vi "Ctor.vi"(8 "error in (no error)":errorcluster, 10 "Object":refnum<class>) -> (0 "error out":errorcluster, 3 "ClassReflector out":refnum<class "ClassReflector.lvclass">)   [LabVIEW 2023, in "ClassReflector.lvclass"]
uses:
  ClassReflector.lvclass
  ClassReflector.lvclass/ClassReflector.ctl
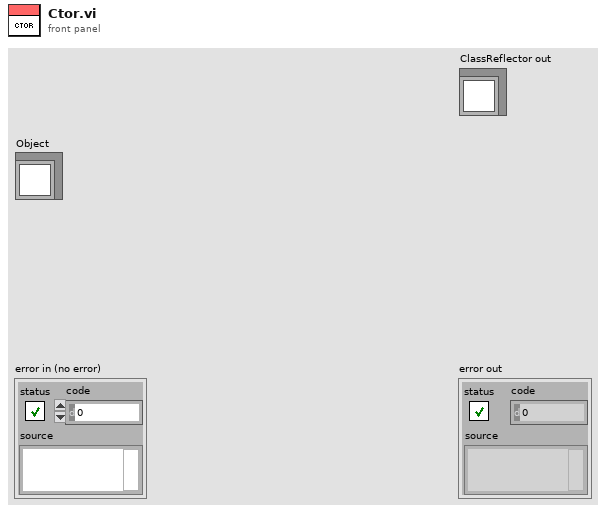
[diagram p1: front panel]
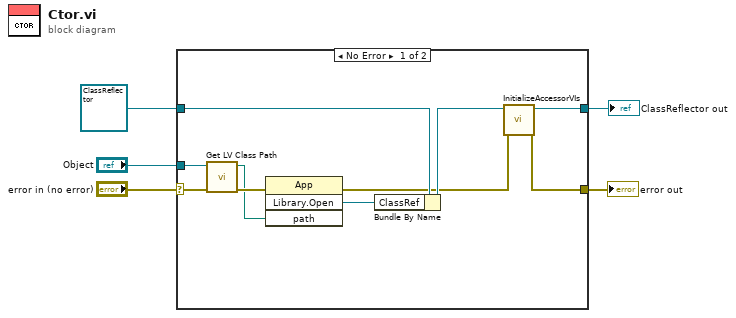
[diagram p0: block diagram]
diagram:
  n1 = case shown="No Error" "error in (no error)" {
    selector: "error in (no error)" -> [w15 w17]
    tunnel: [w6 w17] -> w4
    tunnel: [w8 w16] -> w2
    tunnel: refnum<class "ClassReflector.lvclass"> refnum ("ClassReflector in") -> [w11 w16]
    tunnel: "Object" -> [w13 _]
    frame No Error {
      n2 = call <vilib>:"Get LV Class Path.vi"("error in (no error)"=w15, "object"=w13) -> ("error out"=w14:errorcluster, "class path"=w12:path)  [unwired: 8 in]
      n3 = invoke class="App" method="Library.Open"(error in=w14, "path"=w12) -> (error out=w7:errorcluster, "Open Library"=w10:refnum<vi>)  [unwired: 2 in, 2 out]
      n4 = Bundle By Name(cluster=w11, "ClassRef"=w10) -> (w9:refnum<class "ClassReflector.lvclass">)
      n5 = call "InitializeAccessorVIs.vi"("error in (no error)"=w7, "ClassReflector in"=w9) -> ("error out"=w6:errorcluster, "ClassReflector out"=w8:refnum<class "ClassReflector.lvclass">)  [unwired: 8 in]
    }
    frame Error {
    }
  }
  "error out" <- w4
  "ClassReflector out" <- w2
